vi "FT10_Fornax Ligasure Activate Port Command.vi"(10 "Ligasure Activate":T1, 11 "TCP Network Connection in":refnum<k5>) -> (3 "TCP Network Connection out":refnum<k5>)   [LabVIEW 2024]
doc: "TRUE = Activate Ligasure port via Fornax\nFALSE = Deactivate Ligasure port via Fornax"
uses:
  Controls/Control_Fornax Ligasure Activate Port Bool.ctl
  Controls/Control_Fornax Generator.ctl
  Controls/Control_Fornax Source ID.ctl
  Controls/Control_Fornax Switch ID.ctl
  Controls/Control_Fornax Energy Channel ID.ctl
  Controls/Control_Fornax Switch State.ctl
  Abort Auto Test Global.vi
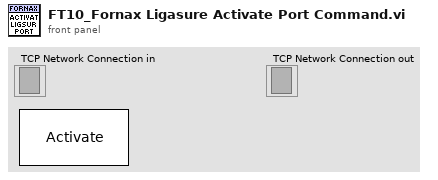
[diagram p1: front panel]
types:
  T1 = typedef "Control_Fornax Ligasure Activate Port Bool.ctl" = bool
  T2 = typedef "Control_Fornax Switch State.ctl" = enum16{"SWITCH_STATE_NULL  ", "SWITCH_STATE_PRESSED  ", "SWITCH_STATE_RELEASED  ", "NUM_SWITCH_STATES  "}
  T3 = typedef "Control_Fornax Energy Channel ID.ctl" = enum16{"EC_MONO_1  ", "EC_BIPOLAR  ", "EC_MONO_2  ", "EC_ADVANCED  ", "EC_ADVANCED_ECUT  ", "EC_ADVANCED_DCUT  ", "EC_SHARED_COAG  ", "EC_INTERNAL_BIP_CAL  "}
  T4 = typedef "Control_Fornax Switch ID.ctl" = enum16{"SWITCH_ID_NONE  ", "SWITCH_ID_CUT  ", "SWITCH_ID_VMODE  ", "SWITCH_ID_COAG  ", "SWITCH_ID_LIGASURE  ", "SWITCH_ID_BIPOLAR  ", "SWITCH_ID_STAPLER_CLOSE  ", "SWITCH_ID_STAPLER_OPEN  ", "SWITCH_ID_CARDIOBLATE_BIPOLAR  ", "SWITCH_ID_CARDIOBLATE_BIPOLAR_TOUCHSCREEN  ", "SWITCH_ID_CARDIOBLATE_MONOPOLAR  ", "SWITCH_ID_CARDIOBLATE_MONOPOLAR_TOUCHSCREEN  ", "SWITCH_ID_ULTRASONIC_BTN1  ", "SWITCH_ID_ULTRASONIC_BTN2  ", "SWITCH_ID_MAX  "}
  T5 = typedef "Control_Fornax Source ID.ctl" = enum16{"SWITCH_SOURCE_UNKNOWN  ", "SWITCH_SOURCE_HANDSWITCH  ", "SWITCH_SOURCE_FOOTSWITCH  ", "SWITCH_SOURCE_AUTO_BIPOLAR  ", "SWITCH_SOURCE_CARDIOBLATE  ", "SWITCH_SOURCE_SCREEN  ", "NUM_SWITCH_SOURCES  "}
  T6 = typedef "Control_Fornax Generator.ctl" = string
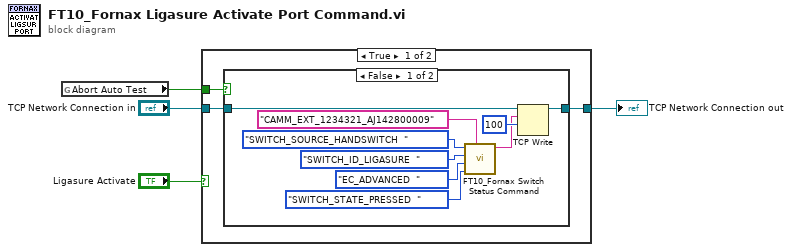
[diagram p0: block diagram]
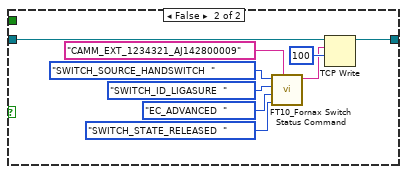
[diagram p3: hidden frame]
diagram:
  n1 = global read "Abort Auto Test Global.vi" "Abort Auto Test"() -> (w1:bool)
  n2 = case shown="True" "Ligasure Activate" {
    tunnel: "TCP Network Connection in" -> [w7 w26]
    tunnel: [w6 w25] -> w4
    tunnel: w1 -> [w5 _]
    frame True {
      n3 = case shown="False" w5 {
        tunnel: w7 -> [w16 w17]
        tunnel: [w15 w17] -> w6
        frame False {
          n4 = call "FT10_Fornax Switch Status Command.vi"("Generator"=T6 "CAMM_EXT_1234321_AJ142800009", "Switch State"=Control_Fornax_Switch_State."SWITCH_STATE_PRESSED  ", "Energy Channel ID"=Control_Fornax_Energy_Channel_ID."EC_ADVANCED  ", "Switch ID"=Control_Fornax_Switch_ID."SWITCH_ID_LIGASURE  ", "Source ID"=Control_Fornax_Source_ID."SWITCH_SOURCE_HANDSWITCH  ") -> ("JSON Command"=w8:string)  [unwired: 6 in]
          n5 = TCP Write(connection ID=w16, data in=w8, 9:100 ("timeout ms (25000)")) -> (connection ID out=w15:refnum<k5>)  [unwired: 1 in, 2 out]
        }
        frame True {
        }
      }
    }
    frame False {
      n6 = call "FT10_Fornax Switch Status Command.vi"("Generator"=T6 "CAMM_EXT_1234321_AJ142800009", "Switch State"=Control_Fornax_Switch_State."SWITCH_STATE_RELEASED  ", "Energy Channel ID"=Control_Fornax_Energy_Channel_ID."EC_ADVANCED  ", "Switch ID"=Control_Fornax_Switch_ID."SWITCH_ID_LIGASURE  ", "Source ID"=Control_Fornax_Source_ID."SWITCH_SOURCE_HANDSWITCH  ") -> ("JSON Command"=w18:string)  [unwired: 6 in]
      n7 = TCP Write(connection ID=w26, data in=w18, 9:100 ("timeout ms (25000)")) -> (connection ID out=w25:refnum<k5>)  [unwired: 1 in, 2 out]
    }
  }
  "TCP Network Connection out" <- w4
